vi "OAT LP Equal Ripple Design.vi"(8 "A stop [dB]":dbl=72.0 format="%.2f", 9 "stopband":dbl=0.25 format="%.2f", 10 "passband":dbl=0.05 format="%.2f", 11 "fs":dbl=1.0 format="%.2f") -> (0 "error":i32, 2 "taps":i32, 3 "filter coefficients":dbl[](array[numeric]) format="%.2f")   [LabVIEW 2017, in "SoundVib_Resampling.lvlib"]
uses:
  <vilib>/addons/Sound and Vibration/Order Analysis/Resample Order Tracking/SoundVib_Resampling.lvlib
  <vilib>/Analysis/NI_AALBase.lvlib
panel:
  in  "debug?":bool
  out "Waveform Graph":T1(graph)
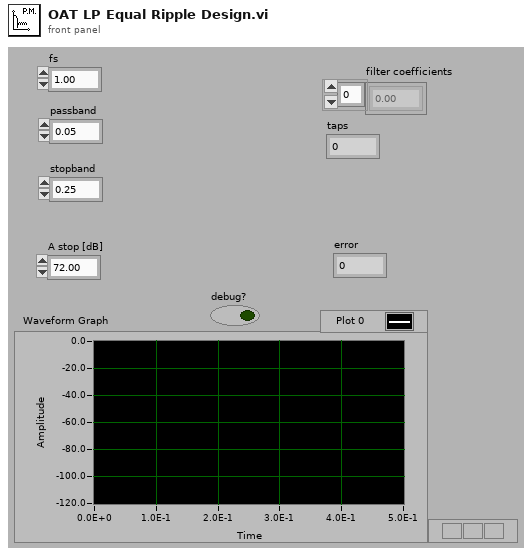
[diagram p1: front panel]
types:
  T1 = cluster{"Lower Freq":dbl, "df":dbl, "amplitude":dbl[]}
  T2 = cluster{"Amplitude":dbl, "Lower Freq":dbl, "Higher Freq":dbl, "Weighted\nRipple":dbl}
  T3 = cluster{"Amplitude":dbl, "Lower Freq":dbl, "Higher Freq":dbl, "Weighted\nRipple":dbl}[]
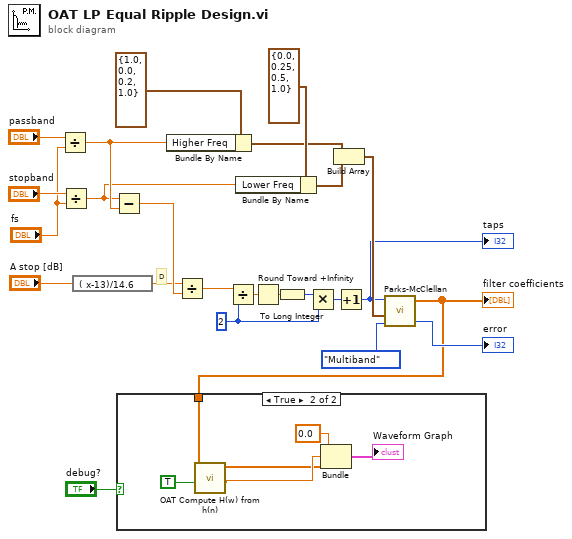
[diagram p0: block diagram]
diagram:
  w4 = 2
  # "D"
  n1 = Divide(x="passband", y="fs") -> (x/y=w16:dbl)
  n2 = Divide(x="stopband", y="fs") -> (x/y=w14:dbl)
  n3 = expression code="( x-13)/14.6"("A stop [dB]") -> (w6:dbl)
  n4 = Subtract(x=w14, y=w16) -> (x-y=w19:dbl)
  n5 = Bundle By Name(cluster=T2 {"Amplitude"=1.0, "Lower Freq"=0.0, "Higher Freq"=0.2, "Weighted\nRipple"=1.0}, "Higher Freq"=w16) -> (w13:T2)
  n6 = Divide(x=w6, y=w19) -> (x/y=w3:dbl)
  n7 = Divide(x=w3, y=w4) -> (x/y=w21:dbl)
  n8 = Bundle By Name(cluster=T2 {"Amplitude"=0.0, "Lower Freq"=0.25, "Higher Freq"=0.5, "Weighted\nRipple"=1.0}, "Lower Freq"=w14) -> (w12:T2)
  n9 = Round Toward +Infinity(x=w21) -> (ceil(x): smallest int >= x=w20:dbl)
  n10 = To Long Integer(number=w20) -> (32bit integer=w18:i32)
  n11 = Multiply(x=w18, y=w4) -> (x*y=w7:i32)
  n12 = Build Array(w13, w12) -> (w11:T3)
  n13 = Increment(x=w7) -> (x+1=w8:i32)
  "taps" <- w8
  n14 = call <vilib>:"Parks-McClellan.vi"("filter type"=enum32{"Multiband", "Differentiator", "Hilbert"}."Multiband", "Band Parameters"=w11, "# of taps"=w8) -> ("error"=→"error":i32, "h"=w1:dbl[])  [unwired: 1 in, 1 out]
  "filter coefficients" <- w1
  n15 = case shown="True" "debug?" {
    tunnel: w1 -> [_ w25]
    frame False {
    }
    frame True {
      n16 = call <vilib>:"OAT Compute H(w) from h(n).vi"("dB on?"=TRUE, "h[n]"=w25) -> ("df"=w29:dbl, "amplitude"=w26:dbl[])  [unwired: 7 in, 1 out]
      n17 = Bundle("Lower Freq"=0.0, "df"=w29, "amplitude"=w26) -> (→"Waveform Graph":T1)  [unwired: 1 in]
    }
  }
